vi "Get PWM Duty.vi"(7 "GPIO":i32, 8 "error in (no error)":errorcluster, 11 "VISA resource name in":refnum<visa-resource-name>) -> (0 "error out":errorcluster, 1 "Duty % (0-1)":sgl, 3 "VISA resource name":refnum<visa-resource-name>)   [LabVIEW 2020, in "CTI-Visa.lvlib"]
uses:
  CTI-Visa.lvlib
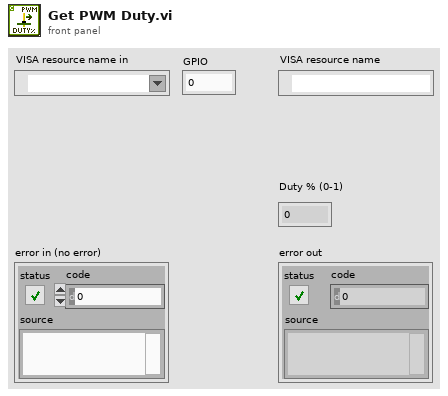
[diagram p1: front panel]
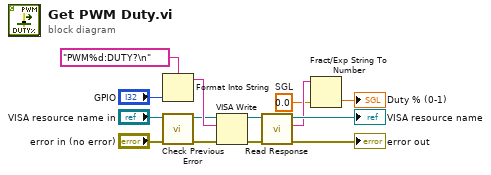
[diagram p0: block diagram]
diagram:
  w2 = sgl 0.0  # SGL
  n1 = Format Into String(format string="PWM%d:DUTY?\n", "GPIO") -> (resulting string=w13:string)  [unwired: 2 in, 1 out]
  n2 = call "Check Previous Error.vi"("error in (no error)"="error in (no error)", "VISA resource name in"="VISA resource name in") -> ("error out"=w7:errorcluster, "VISA resource name"=w9:refnum<visa-resource-name>)  [unwired: 8 in]
  n3 = VISA Write(VISA resource name=w9, write buffer=w13, error in (no error)=w7) -> (VISA resource name out=w11:refnum<visa-resource-name>, error out=w5:errorcluster)  [unwired: 1 out]
  n4 = call "Read Response.vi"("error in (no error)"=w5, "VISA resource name in"=w11) -> ("error out"=→"error out":errorcluster, "Response"=w3:string, "VISA resource name"=→"VISA resource name":refnum<visa-resource-name>)  [unwired: 7 in]
  n5 = Fract/Exp String To Number(string=w3, default (0 dbl)=w2) -> (number=→"Duty % (0-1)":sgl)  [unwired: 2 in, 1 out]
